vi "format date and time.vi"   [LabVIEW 2023, in "Reusable Library.lvlib"]
uses:
  Reusable Library.lvlib
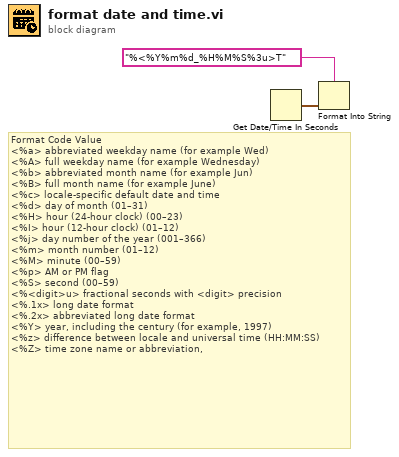
[diagram p0: block diagram]
diagram:
  # "Format Code\tValue\n<%a>\tabbreviated weekday name (for example Wed)\n<%A>\tfull weekday name (for example Wednesday)\n<%b>\tabbreviated month name (for example Jun)\n<%B>\tfull month name (for example June)\n<%c>\tlocale-specific default date and time\n<%d>\tday of month (01–31)\n<%H>\thour (24-hour clock) (00–23)\n<%I>\thour (12-hour clock) (01–12)\n<%j>\tday number of the year (001–366)\n<%m>\tmonth number (01–12)\n<%M>\tminute (00–59)\n<%p>\tAM or PM flag\n<%S>\tsecond (00–59)\n<%<digit>u>\tfractional seconds with <digit> precision\n<%.1x>\tlong date format\n<%.2x>\tabbreviated long date format\n<%Y>\tyear, including the century (for example, 1997)\n<%z>\tdifference between locale and universal time (HH:MM:SS)\n<%Z>\ttime zone name or abbreviation,"
  n1 = Get Date/Time In Seconds() -> (seconds since 1Jan1904=w1:timestamp)
  n2 = Format Into String(format string="%<%Y%m%d_%H%M%S%3u>T", w1) -> ()  [unwired: 2 in, 2 out]
